vi "Go to Goal with Orientation.vi"(10 "Goal Frame (World)":cluster{"X":sgl, "Y":sgl, "Theta":dbl}, 11 "Robot Frame (World)":cluster{"X":sgl, "Y":sgl, "Theta":dbl}) -> (2 "Goal Arrive?":bool, 3 "Frame Velocity":dbl[](array[numeric]))   [LabVIEW 2016]
uses:
  <vilib>/Analysis/coordinate.llb/Angle Units.ctl
  <vilib>/Analysis/coordinate.llb/Angle Range (Degree).ctl
  <vilib>/Analysis/coordinate.llb/Wrap Angle (scalar).vi
  <vilib>/Analysis/NI_AAL_Angle.lvlib
panel:
  out "s? t:f":dbl
  out "alpha":dbl
  in  "K3 (have to be negative)":dbl=-1.5
  in  "K2":dbl=6.0
  in  "K1":dbl=1.5
  out "rho":sgl
  out "delta Y":sgl
  out "delta X":sgl
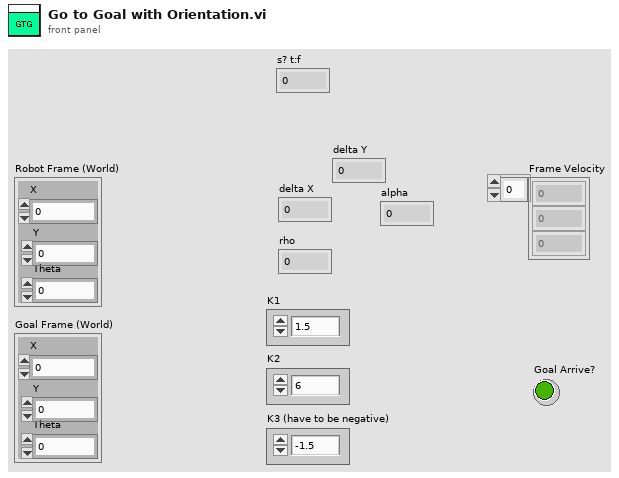
[diagram p1: front panel]
types:
  T1 = typedef "NI_AAL_Angle.lvlib/Angle Range (Degree).ctl" = u16
  T2 = typedef "NI_AAL_Angle.lvlib/Angle Units.ctl" = i32
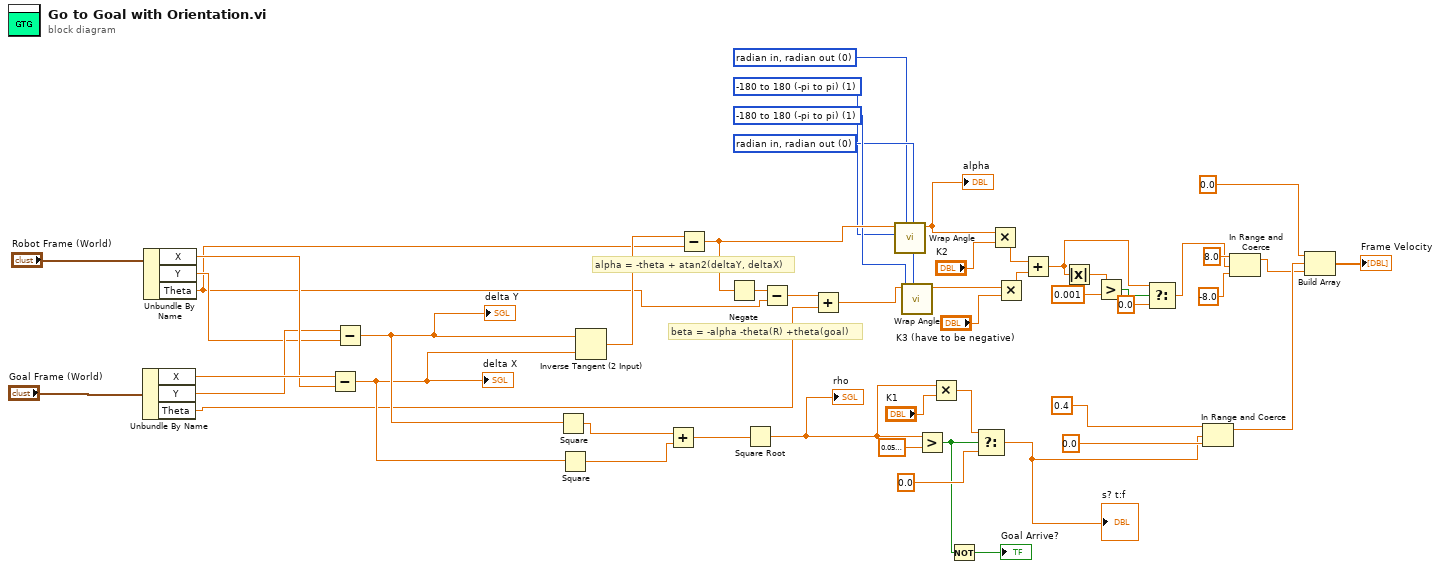
[diagram p0: block diagram]
diagram:
  w33 = T1 1 items=["none", "-180 to 180 (-pi to pi)", "0 to 360 (0 to 2pi)"] ("angle range")
  w34 = T2 0 items=["radian in, radian out", "radian in, degree out", "degree in, degree out", "degree in, radian out"] ("angle units")
  w35 = T2 0 items=["radian in, radian out", "radian in, degree out", "degree in, degree out", "degree in, radian out"] ("angle units")
  w36 = T1 1 items=["none", "-180 to 180 (-pi to pi)", "0 to 360 (0 to 2pi)"] ("angle range")
  # "beta = -alpha -theta(R) +theta(goal)"
  # "alpha = -theta + atan2(deltaY, deltaX)"
  n1 = Unbundle By Name("Goal Frame (World)") -> ("X"=w48:sgl, "Y"=w46:sgl, "Theta"=w10:dbl)
  n2 = Unbundle By Name("Robot Frame (World)") -> ("X"=w47:sgl, "Y"=w45:sgl, "Theta"=w11:dbl)
  n3 = Subtract(x=w48, y=w47) -> (x-y=w41:sgl)
  "delta X" <- w41
  n4 = Subtract(x=w46, y=w45) -> (x-y=w42:sgl)
  "delta Y" <- w42
  n5 = Square(x=w42) -> (x^2=w40:sgl)
  n6 = Square(x=w41) -> (x^2=w39:sgl)
  n7 = Inverse Tangent (2 Input)(1:w41, 2:w42) -> (0:w44:sgl)
  n8 = Add(x=w40, y=w39) -> (x+y=w38:sgl)
  n9 = Subtract(x=w44, y=w11) -> (x-y=w37:dbl)
  n10 = Negate(x=w37) -> (-x=w43:dbl)
  n11 = Square Root(x=w38) -> (sqrt(x)=w27:sgl)
  "rho" <- w27
  n12 = Subtract(x=w43, y=w11) -> (x-y=w9:dbl)
  n13 = Add(x=w9, y=w10) -> (x+y=w8:dbl)
  n14 = call-poly <vilib>:"Wrap Angle.vi"("angle units"=w34, "angle range"=w33, "angle in"=w37) -> ("angle out"=w32:dbl)  [unwired: 7 in, 1 out]
  "alpha" <- w32
  n15 = call-poly <vilib>:"Wrap Angle.vi"("angle units"=w35, "angle range"=w36, "angle in"=w8) -> ("angle out"=w31:dbl)  [unwired: 7 in, 1 out]
  n16 = Greater?(x=w27, y=sgl 0.05) -> (0:w19:bool)
  n17 = Multiply(x=w27, y="K1") -> (x*y=w26:dbl)
  n18 = Not(x=w19) -> (.not. x?=→"Goal Arrive?":bool)
  n19 = Select(t=w26, s=w19, f=sgl 0.0) -> (s? t:f=w1:dbl)
  "s? t:f" <- w1
  n20 = Multiply(x=w32, y="K2") -> (x*y=w29:dbl)
  n21 = Multiply(x=w31, y="K3 (have to be negative)") -> (x*y=w30:dbl)
  n22 = Add(x=w29, y=w30) -> (x+y=w5:dbl)
  n23 = Absolute Value(x=w5) -> (abs(x)=w2:dbl)
  n24 = Greater?(x=w2, y=0.001) -> (0:w6:bool)
  n25 = Select(t=w5, s=w6, f=0.0) -> (s? t:f=w3:dbl)
  n26 = In Range and Coerce(upper limit=0.4, x=w1, lower limit=0.0) -> (coerced(x)=w15:dbl)  [unwired: 1 out]
  n27 = In Range and Coerce(upper limit=8.0, x=w3, lower limit=-8.0) -> (coerced(x)=w12:dbl)  [unwired: 1 out]
  n28 = Build Array(0.0 ("index"), w15, w12) -> (→"Frame Velocity":dbl[])
